vi "Update Caller.vi"(8 "error in (no error)":cluster{"状态":bool, "代码":i32, "源":string} caption="错误输入（无错误）", 9 "新值":cluster{"风扇A":T1, "风扇B":T1}, 10 "原值":cluster{"风扇A":T1, "风扇B":T1}, 11 "双风扇":refnum<class "Dual Fan.lvclass">) -> (0 "error out":cluster{"状态":bool, "代码":i32, "源":string} caption="错误输出")   [LabVIEW 2015, in "Dual Fan.lvlib" / "Dual Fan.lvclass"]
uses:
  Dual Fan.lvclass
  Fan Info.ctl
  <vilib>/ActorFramework/Actor/Actor.lvclass/Actor.ctl
  Dual Fan.lvclass/Dual Fan.ctl
  Update Fan Status Msg/Update Fan Status Msg.lvclass/Update Fan Status Msg.ctl
  <vilib>/ActorFramework/Message Enqueuer/Message Enqueuer.lvclass/Message Enqueuer.ctl
  <vilib>/ActorFramework/Message Enqueuer/Enqueue.vi
  <vilib>/ActorFramework/Message Priority Queue/Priority Enqueue.vi
  <vilib>/ActorFramework/Actor/Actor.lvclass
  Update Fan Status Msg/Update Fan Status Msg.lvclass
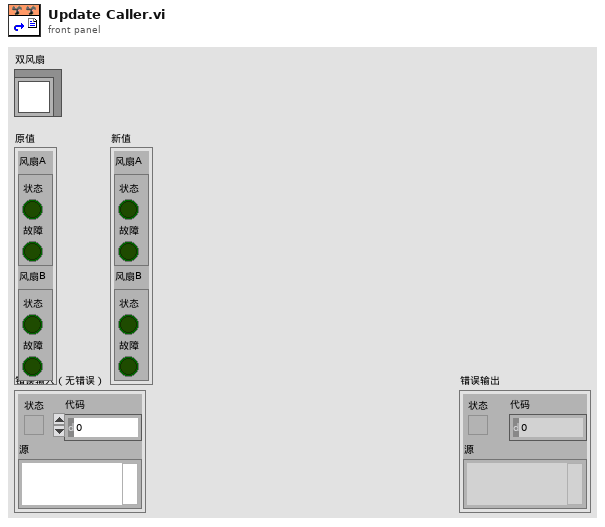
[diagram p1: front panel]
types:
  T1 = typedef "Dual Fan.lvlib/Dual Fan.lvclass/Fan Info.ctl" = cluster{"状态":bool, "故障":bool}
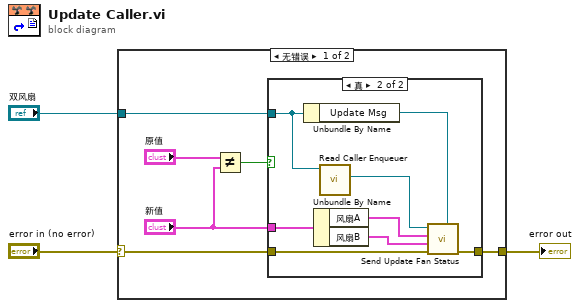
[diagram p0: block diagram]
diagram:
  n1 = case shown="无错误" "error in (no error)" {
    selector: "error in (no error)" -> [w8 w19]
    tunnel: [w7 w19] -> w2
    tunnel: "双风扇" -> [w9 _]
    frame No Error {
      n2 = Not Equal?(x="原值", y="新值") -> (x != y?=w5:bool)
      n3 = case shown="真" w5 {
        tunnel: w9 -> [_ w18]
        tunnel: w8 -> [w10 w15]
        tunnel: [w10 w14] -> w7
        tunnel: "新值" -> [_ w13]
        frame False {
        }
        frame True {
          n4 = Unbundle By Name(w18) -> ("Update Msg"=w16:refnum<class "Update Fan Status Msg.lvclass">)
          n5 = Unbundle By Name(w13) -> ("风扇A"=w12:T1, "风扇B"=w11:T1)
          n6 = call <vilib>:"Read Caller Enqueuer.vi"("Actor"=w18) -> ("Caller Enqueuer"=w17:refnum<class "Message Enqueuer.lvclass">)  [unwired: 10 in]
          n7 = call "Send Update Fan Status.vi"("更新消息对象"=w16, "error in (no error)"=w15, "风扇B"=w11, "风扇A"=w12, "消息待入队列"=w17) -> ("error out"=w14:cluster{"状态":bool, "代码":i32, "源":string})  [unwired: 6 in]
        }
      }
    }
    frame Error {
    }
  }
  "error out" <- w2
